vi "Spy Check Process Messages Received.vi"(8 "error in (no error)":errorcluster, 11 "Mock Process In":refnum<class "Mock Process.lvclass">) -> (0 "error out":errorcluster, 1 "Messages":string[](array[string]), 2 "Messages received?":bool, 3 "Mock Process Out":refnum<class "Mock Process.lvclass">)   [LabVIEW 2020, in "Mock Process.lvclass"]
uses:
  Mock Process.lvclass
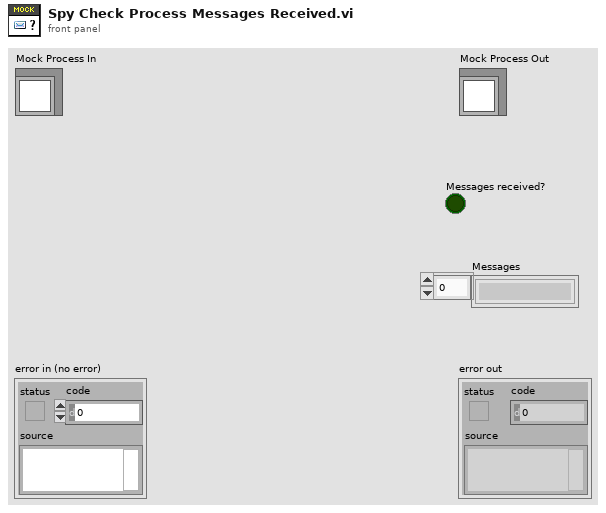
[diagram p1: front panel]
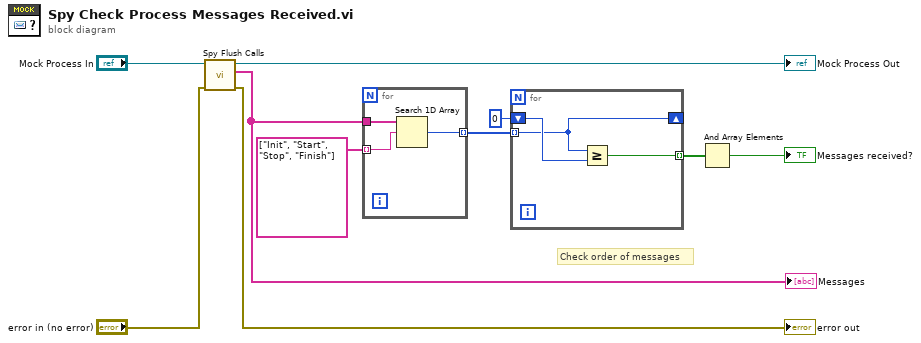
[diagram p0: block diagram]
diagram:
  # "Check order of messages"
  n1 = call "Spy Flush Calls.vi"("error in (no error)"="error in (no error)", "Mock Process In"="Mock Process In") -> ("error out"=→"error out":errorcluster, "Message"=w1:string[], "Mock Process Out"=→"Mock Process Out":refnum<class "Mock Process.lvclass">)  [unwired: 6 in, 1 out]
  "Messages" <- w1
  n2 = for {
    tunnel: w1 -> [w13]
    tunnel: string[] ["Init", "Start", "Stop", "Finish"] ("element") -> [w12] mode=indexing
    tunnel: [w11] -> w5 mode=indexing
    n3 = Search 1D Array(1D array=w13, element=w12) -> (index of element=w11:i32)  [unwired: 1 in]
  }
  n4 = for {
    tunnel: w5 -> [w14] mode=indexing
    shift-right: [w14] -> _
    shift-left: 0 ("index of element") -> [w16]
    tunnel: [w15] -> w3 mode=indexing
    n5 = Greater Or Equal?(x=w14, y=w16) -> (x >= y?=w15:bool)
  }
  n6 = And Array Elements(Boolean array=w3) -> (logical AND=→"Messages received?":bool)
